vi "GetPiece.vi"(1 "PieceIndex":i32, 2 "Board":i32[][](array[numeric])=[[-3, -5, -4, -1, -2, -4, -5, -3], [-6, -6, -6, -6, -6, -6, -6, -6], [0, 0, 0, 0, 0, 0, 0, 0], [0, 0, 0, 0, 0, 0, 0, 0], [0, 0, 0, 0, 0, 0, 0, 0], [0, 0, 0, 0, 0, 0, 0, 0], [6, 6, 6, 6, 6, 6, 6, 6], [3, 5, 4, 1, 2, 4, 5, 3]]) -> (0 "Piece":i32)   [LabVIEW 2014]
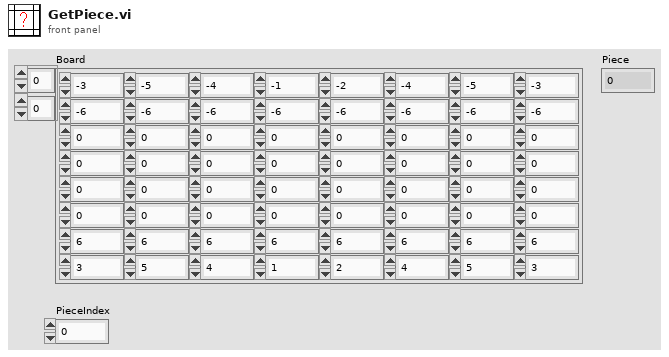
[diagram p1: front panel]
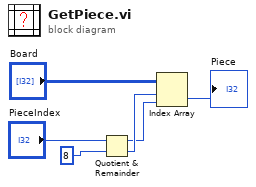
[diagram p0: block diagram]
diagram:
  n1 = Quotient & Remainder(x="PieceIndex", y=8) -> (x-y*floor(x/y)=w3:i32, floor(x/y)=w4:i32)
  n2 = Index Array(array="Board", index (row)=w4, index (col)=w3) -> (element=→"Piece":i32)
